vi "USRP Sampling test.vi"() -> ()   [LabVIEW 2014]
panel:
  out "output":dbl[][](array[numeric])
  out "last value":dbl
  out "error out":errorcluster
  in  "Wifi Channel":i32=3
  in  "parameter":T1={"Method"=enum."Binary", "offset"=0, "threshold"=1.0, "step"=1.0}
  in  "setup para":T2={"Active Antenna"="RX2", "Carrier Frequency"=0.0, "IQ Rate"=0.0, "Gain"=0.0}
  in  "device names":refnum<k15>="192.168.10.2"
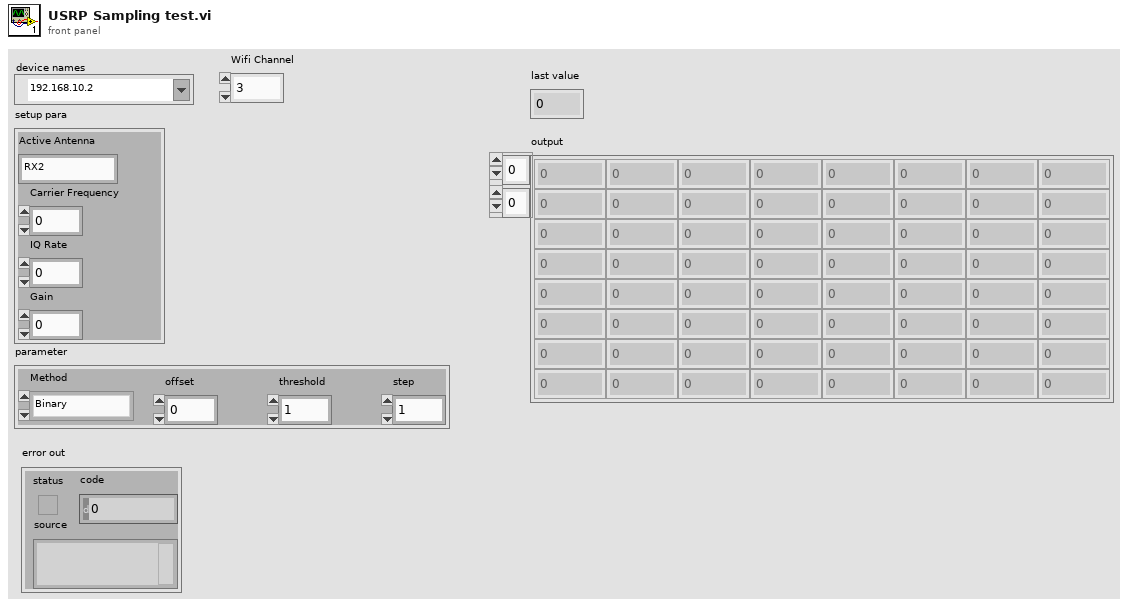
[diagram p1: front panel]
types:
  T1 = cluster{"Method":enum16{"Binary", "Uniform"}, "offset":i32, "threshold":dbl, "step":dbl}
  T2 = cluster{"Active Antenna":string, "Carrier Frequency":dbl, "IQ Rate":dbl, "Gain":dbl}
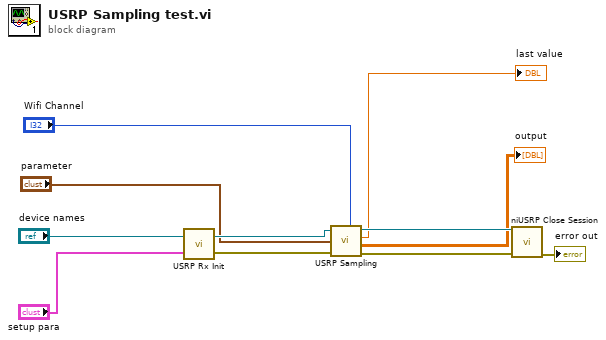
[diagram p0: block diagram]
diagram:
  n1 = call "USRP Rx Init.vi"("setup para"="setup para", "device names"="device names") -> ("error out"=w11:errorcluster, "session handle out"=w10:refnum<k15>)
  n2 = call "USRP Sampling.vi"("Wifi Channel"="Wifi Channel", "error in"=w11, "parameter"="parameter", "session handle in"=w10) -> ("error out"=w4:errorcluster, "output"=→"output":dbl[][], "last value"=→"last value":dbl, "session handle out"=w5:refnum<k15>)
  n3 = call <instrlib>:"niUSRP Close Session.vi"("session handle"=w5, "error in (no error)"=w4) -> ("error out"=→"error out":errorcluster)  [unwired: 13 in]
